vi "Inline Start.vi"(7 "Command":T1, 8 "error in (no error)":errorcluster, 10 "Dispatcher Interface in":refnum<class "Dispatcher Interface.lvclass">, 11 "Plugin Timing Group in":refnum<class "Scheduler Plugin Bundle.lvclass">) -> (0 "error out":errorcluster, 2 "Dispatcher Interface out":refnum<class "Dispatcher Interface.lvclass">, 3 "Plugin Timing Group out":refnum<class "Scheduler Plugin Bundle.lvclass">)   [LabVIEW 2017, in "DSF Core.lvlib" / "Scheduler Plugin Bundle.lvclass"]
uses:
  Scheduler/Scheduler Plugin Bundle.lvclass
  Interfaces/Dispatcher/Dispatcher Interface.lvclass
  Interfaces/Dispatcher/Command.ctl
  Scheduler/Scheduler Plugin Bundle.lvclass/Scheduler Plugin Bundle.ctl
  Scheduler/Scheduler Transfer Group Bundle.lvclass
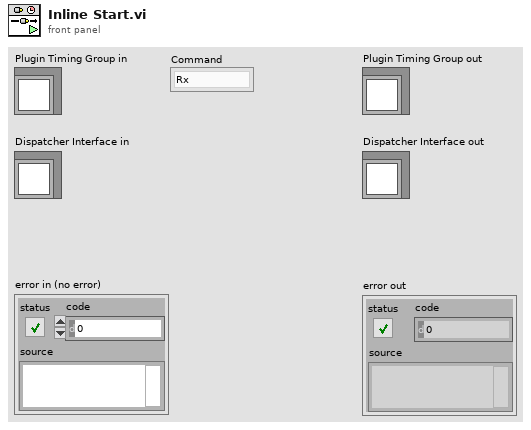
[diagram p1: front panel]
types:
  T1 = typedef "DSF Core.lvlib/Dispatcher Interface.lvclass/Command.ctl" = enum8{"Rx", "Tx", "Shutdown"}
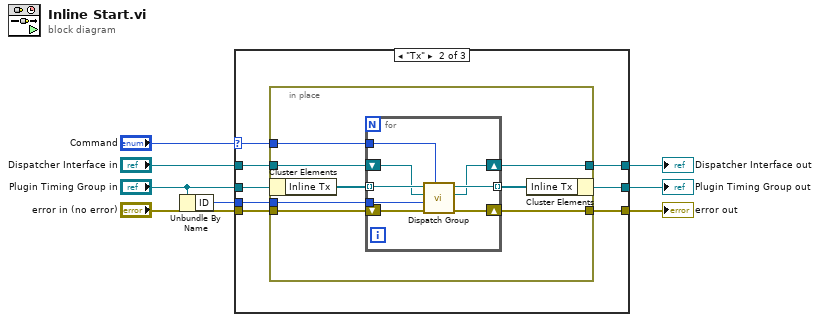
[diagram p0: block diagram]
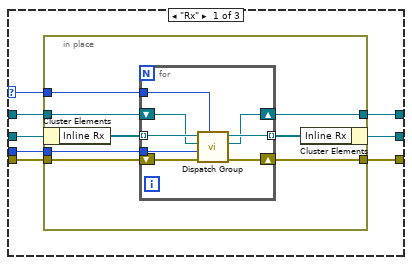
[diagram p2: hidden frame]
diagram:
  n1 = Unbundle By Name("Plugin Timing Group in") -> ("ID"=w2:i32)
  n2 = case shown="\"Tx\"" "Command" {
    selector: "Command" -> [w9 w33 _]
    tunnel: [w16 w40 w58] -> w8
    tunnel: "Dispatcher Interface in" -> [w15 w39 w59]
    tunnel: [w14 w38 w59] -> w6
    tunnel: "error in (no error)" -> [w13 w37 w57]
    tunnel: [w12 w36 w57] -> w4
    tunnel: "Plugin Timing Group in" -> [w11 w35 w58]
    tunnel: w2 -> [w10 w34 _]
    frame "Rx" {
      n3 = in-place {
        in-place-border: w15 -> [w23]
        in-place-border: [w22] -> w14
        in-place-border: [w21] -> w12
        in-place-border: w13 -> [w20]
        in-place-border: w10 -> [w19]
        in-place-border: w9 -> [w17]
        n4 = in-place-cluster #1(w11) -> ("Inline Rx"=w24:refnum<class "Scheduler Transfer Group Bundle.lvclass">[])
        n5 = for {
          tunnel: w24 -> [w32] mode=indexing
          shift-right: [w26] -> w22
          shift-left: w23 -> [w29]
          shift-right: [w30] -> w21
          shift-left: w20 -> [w31]
          tunnel: w19 -> [w27]
          tunnel: [w28] -> w18 mode=indexing
          tunnel: w17 -> [w25]
          n6 = call "Dispatch Group.vi"("Command"=w25, "error in (no error)"=w31, "Plugin ID"=w27, "Dispatcher Interface in"=w29, "Scheduler Transfer Group Bundle in"=w32) -> ("error out"=w30:errorcluster, "Dispatcher Interface out"=w26:refnum<class "Dispatcher Interface.lvclass">, "Scheduler Transfer Group Bundle out"=w28:refnum<class "Scheduler Transfer Group Bundle.lvclass">)  [unwired: 4 in]
        }
        n7 = in-place-cluster #1("Inline Rx"=w18) -> (w16:refnum<class "Scheduler Plugin Bundle.lvclass">)
      }
    }
    frame "Tx" {
      n8 = in-place {
        in-place-border: w39 -> [w47]
        in-place-border: [w46] -> w38
        in-place-border: [w45] -> w36
        in-place-border: w37 -> [w44]
        in-place-border: w34 -> [w43]
        in-place-border: w33 -> [w41]
        n9 = in-place-cluster #2(w35) -> ("Inline Tx"=w48:refnum<class "Scheduler Transfer Group Bundle.lvclass">[])
        n10 = for {
          tunnel: w48 -> [w56] mode=indexing
          shift-right: [w50] -> w46
          shift-left: w47 -> [w53]
          shift-right: [w54] -> w45
          shift-left: w44 -> [w55]
          tunnel: w43 -> [w51]
          tunnel: [w52] -> w42 mode=indexing
          tunnel: w41 -> [w49]
          n11 = call "Dispatch Group.vi"("Command"=w49, "error in (no error)"=w55, "Plugin ID"=w51, "Dispatcher Interface in"=w53, "Scheduler Transfer Group Bundle in"=w56) -> ("error out"=w54:errorcluster, "Dispatcher Interface out"=w50:refnum<class "Dispatcher Interface.lvclass">, "Scheduler Transfer Group Bundle out"=w52:refnum<class "Scheduler Transfer Group Bundle.lvclass">)  [unwired: 4 in]
        }
        n12 = in-place-cluster #2("Inline Tx"=w42) -> (w40:refnum<class "Scheduler Plugin Bundle.lvclass">)
      }
    }
    frame "Shutdown", Default {
    }
  }
  "Plugin Timing Group out" <- w8
  "Dispatcher Interface out" <- w6
  "error out" <- w4
